vi "set_channel_offsets.vi"(8 "error in (no error)":errorcluster, 10 "pixel values cluster":T1, 11 "FPGAWrapperDL090211Galvo in":refnum<class "FPGAWrapperDL090211Galvo.lvclass">) -> (0 "error out":errorcluster, 3 "FPGAWrapperDL090211Galvo out":refnum<class "FPGAWrapperDL090211Galvo.lvclass">)   [LabVIEW 2010, in "FPGAWrapperDL090211Galvo.lvclass"]
uses:
  FPGAWrapperDL090211Galvo.lvclass
  common_typedefs/channels_cluster.ctl
  FPGAWrapperDL090211Galvo.lvclass/FPGAWrapperDL090211Galvo.ctl
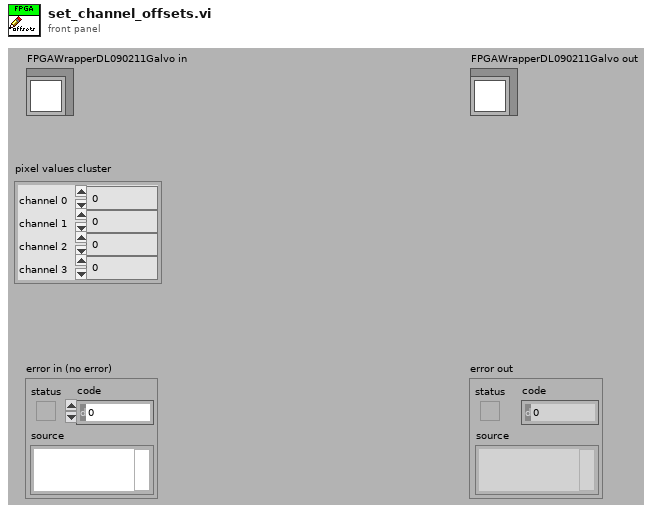
[diagram p1: front panel]
types:
  T1 = typedef "channels_cluster.ctl" = cluster{"channel 0":u32, "channel 1":u32, "channel 2":u32, "channel 3":u32}
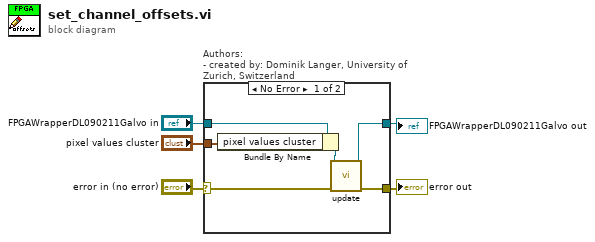
[diagram p0: block diagram]
diagram:
  n1 = case "Authors: \n- created by: Dominik Langer, University of Zurich, Switzerland" shown="No Error" "error in (no error)" {
    selector: "error in (no error)" -> [w9 w13]
    tunnel: [w6 w12] -> w2
    tunnel: [w8 w13] -> w1
    tunnel: "FPGAWrapperDL090211Galvo in" -> [w11 w12]
    tunnel: "pixel values cluster" -> [w10 _]
    frame No Error {
      n2 = Bundle By Name(cluster=w11, "pixel values cluster"=w10) -> (w7:refnum<class "FPGAWrapperDL090211Galvo.lvclass">)
      n3 = call-dynamic "update.vi"("error in (no error)"=w9, "FPGAWrapperDL120115Galvo in"=w7) -> ("error out"=w8:errorcluster, "FPGAWrapperDL120115Galvo out"=w6:refnum<class "FPGAWrapperDL090211Galvo.lvclass">)  [unwired: 8 in]
    }
    frame Error {
    }
  }
  "error out" <- w1
  "FPGAWrapperDL090211Galvo out" <- w2
